vi "题目1.vi"() -> ()   [LabVIEW 2017]
uses:
  <vilib>/measure/NI_MABase.lvlib
panel:
  in  "布尔":bool
  out "波形图 2":waveform(dbl)(graph)
  out "波形图":waveform(dbl)(graph)
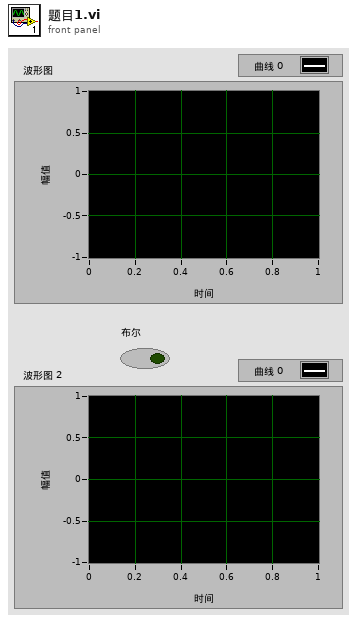
[diagram p1: front panel]
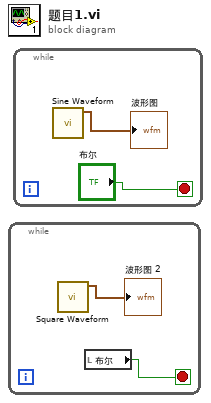
[diagram p0: block diagram]
diagram:
  n1 = while {
    stop <- w1 stop-if-true
    n2 = call <vilib>:"Square Waveform.vi"() -> ("signal out"=→"波形图 2":waveform(dbl))  [unwired: 10 in, 1 out]
    n3 = local read "布尔"() -> (w1:bool)
  }
  n4 = while {
    stop <- "布尔" stop-if-true
    n5 = call <vilib>:"Sine Waveform.vi"() -> ("signal out"=→"波形图":waveform(dbl))  [unwired: 10 in, 1 out]
  }
